vi "Disable Selection.vi"(8 "error in (no error)":errorcluster, 10 "Disable?":bool, 11 "Scheduler in":refnum<class "Scheduler.lvclass">) -> (0 "error out":errorcluster, 3 "Scheduler out":refnum<class "Scheduler.lvclass">)   [LabVIEW 2020, in "Scheduler.lvlib" / "Scheduler.lvclass"]
uses:
  Scheduler.lvclass
  C:/Users/marco/Documents/GitHub_Lab/TALOS/talos/Father of all uServices/Father of all uServices/Father of all uServices.lvclass
  Ancestor/Ancestor/Ancestor.lvclass/Ancestor.ctl
  Support VIs/Generate Error.vi
  FGV/Error Memory/Get Error Description.vi
  Support VIs/Get PC name.vi
  Ancestor/Ancestor/Read ID.vi
  Support VIs/Get Class Name.vi
  <vilib>/Utility/error.llb/Clear Errors.vi
  FGV/Error Memory/Error Memory Core.vi
  <vilib>/AdvancedString/Delimited String to 1D String Array.vi
  Support VIs/Circus Root Path.vi
  FGV/Error Memory/Error Crt Lvl checker.vi
  FGV/Error Memory/Error Memory Core.vi/40c8088d-b597-4017-91af-faa98e00292e.vi
  FGV/Error Memory/Error Memory Core.vi/d4a3ab98-063c-4e44-b43d-fbdcfe6c2be2.vi
  Support VIs/Global Memory.vi
  <vilib>/Utility/LVClass/Get LV Class Name.vi
  Support VIs/Is in Packed Library.vi
  Support VIs/TALOS Root path.vi
  Support VIs/Read CSV worksheet.vi
  Support VIs/Global Constants.vi
  <vilib>/Utility/error.llb/General Error Handler.vi
  Support VIs/Error Log.vi
  Ancestor/Ancestor/Ancestor.lvclass
  <vilib>/Comparison/Equal/Equal Functor/Equal Functor.lvclass
  TALOS.lvlib
  Father of all uServices/Father of all uServices/Father of all uServices.lvclass
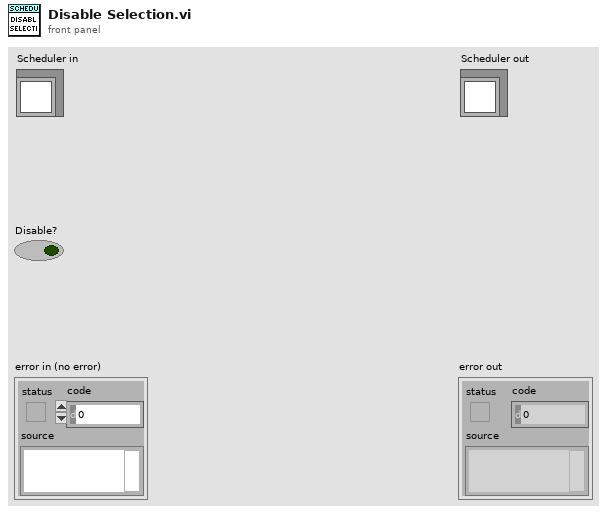
[diagram p1: front panel]
types:
  T1 = enum8{"Enabled", "Disabled", "Disabled and Grayed Out"}
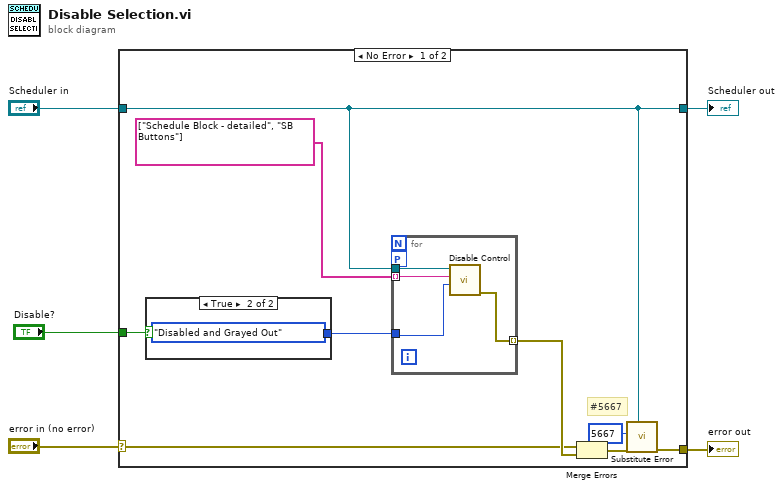
[diagram p0: block diagram]
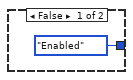
[diagram p2: hidden frame]
diagram:
  n1 = case shown="No Error" "error in (no error)" {
    selector: "error in (no error)" -> [w9 w22]
    tunnel: [w11 w22] -> w4
    tunnel: [w7 w21] -> w2
    tunnel: "Scheduler in" -> [w7 w21]
    tunnel: "Disable?" -> [w14 _]
    frame No Error {
      # "#5667"
      n2 = case shown="True" w14 {
        tunnel: [T1."Enabled" ("Disabled") T1."Disabled and Grayed Out" ("Disabled")] -> w13
        frame False {
        }
        frame True {
        }
      }
      n3 = for {
        tunnel: w13 -> [w18]
        tunnel: string[] ["Schedule Block - detailed", "SB Buttons"] -> [w17] mode=indexing
        tunnel: [w15] -> w10 mode=indexing
        tunnel: w7 -> [w16]
        workers-P: _ -> [_]
        n4 = call "Disable Control.vi"("Disabled"=w18, "FP Item Name"=w17, "Father of all uServices in"=w16) -> ("error out"=w15:errorcluster)  [unwired: 7 in, 1 out]
      }
      n5 = Merge Errors(w9, w10) -> (w8:errorcluster)
      n6 = call "Substitute Error.vi"("LabVIEW Object"=w7, "error in (no error)"=w8, "Error Code"=5667) -> ("error out"=w11:errorcluster)  [unwired: 8 in]
    }
    frame Error {
    }
  }
  "error out" <- w4
  "Scheduler out" <- w2
